vi "TCP Connection Manager (By Reference).vi"(0 "connection manager ref in":T1, 5 "connection in":T3, 7 "index":i32, 9 "method":T5, 11 "error in":errorcluster, 12 "properties in":T2) -> (3 "all properties":T2[](array[typedef]), 4 "connection manager ref out":T1, 6 "connection out":T3, 8 "all connections":T3[](array[typedef]), 10 "number of connections":i32, 14 "properties out":T2, 15 "error out":errorcluster)   [LabVIEW 2015, in "NI STM.lvlib"]
doc: "Copyright 2015, 2016, 2017 National Instruments Corporation\n\nLicensed under the Apache License, Version 2.0 (the \"License\"); you may not use this file except in compliance with the License.\n\n You may obtain a copy of the License at\n\n http://www.apache.org/licenses/LICENSE-2.0\n\nUnless required by applicable law or agreed to in writing, software distributed under the License is distributed on an \"AS IS\" BASIS, WITHOUT WARRANTIES OR CONDITIONS OF ANY KIND, either express or implied.\n\nSee the License for the specific language governing permissions and limitations under the License."
uses:
  <vilib>/NI/STM/NI STM.lvlib
  <vilib>/NI/STM/Connection Manager/TCP/TCP Connection Method.ctl
  <vilib>/NI/STM/TCP/TCP Connection Info.ctl
  <vilib>/NI/STM/SubVIs/MetaDataElement.ctl
  <vilib>/NI/STM/Connection Manager/TCP/TCP Connection Properties.ctl
  <vilib>/NI/STM/Connection Manager/TCP/Advanced/TCP Connection Manager Reference.ctl
  <vilib>/NI/STM/Connection Manager/TCP/Advanced/TCP Connection Manager State Variables.ctl
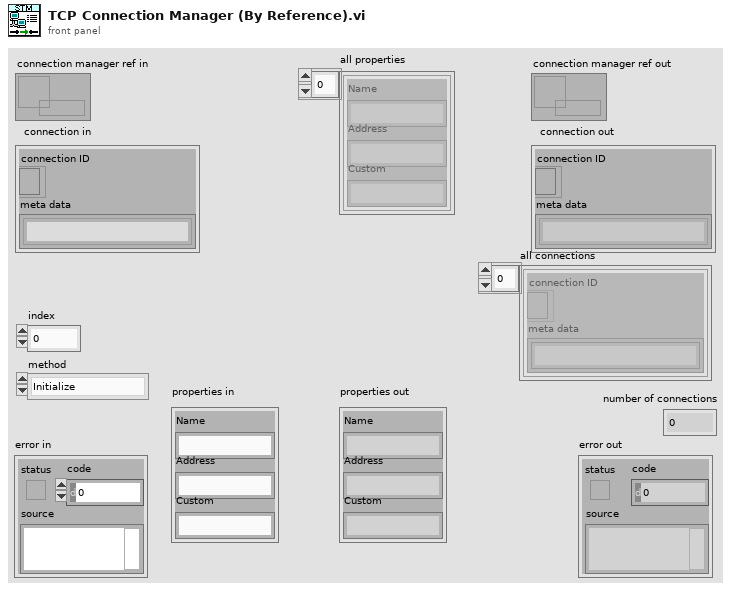
[diagram p1: front panel]
types:
  T1 = typedef "NI STM.lvlib/TCP Connection Manager Reference.ctl" = refnum<data-value>
  T2 = typedef "NI STM.lvlib/TCP Connection Properties.ctl" = cluster{"Name":string, "Address":string, "Custom":string}
  T3 = typedef "NI STM.lvlib/TCP Connection Info.ctl" = cluster{"connection ID":refnum<k5>, "meta data":T4[]}
  T4 = typedef "NI STM.lvlib/MetaDataElement.ctl" = string
  T5 = typedef "NI STM.lvlib/TCP Connection Method.ctl" = enum16{"Initialize", "Add Connection", "Set Properties", "Get Connection(s)", "Remove Connection", "Remove All Connections", "Get Connection Count"}
  T6 = typedef "NI STM.lvlib/TCP Connection Manager State Variables.ctl" = cluster{"Connections":T3[], "Properties":T2[]}
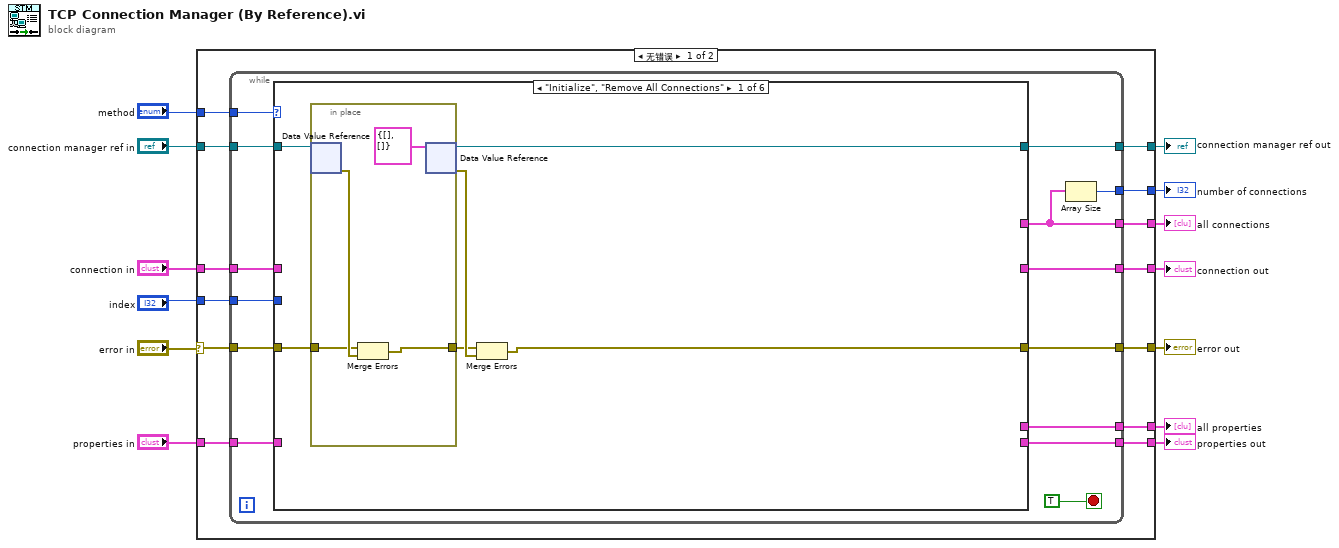
[diagram p0: block diagram]
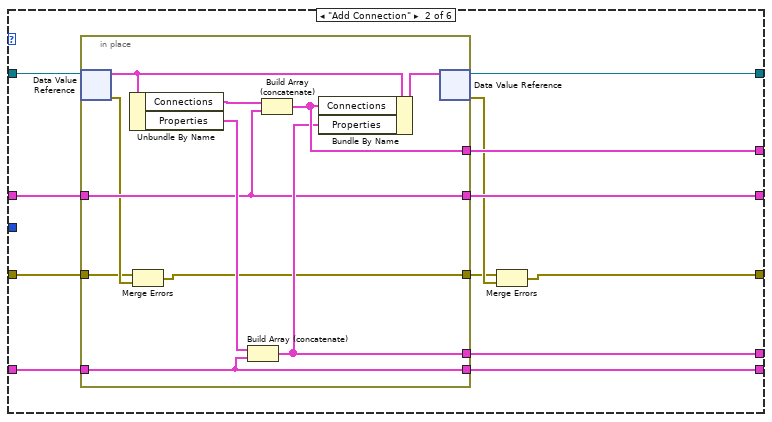
[diagram p2: hidden frame]
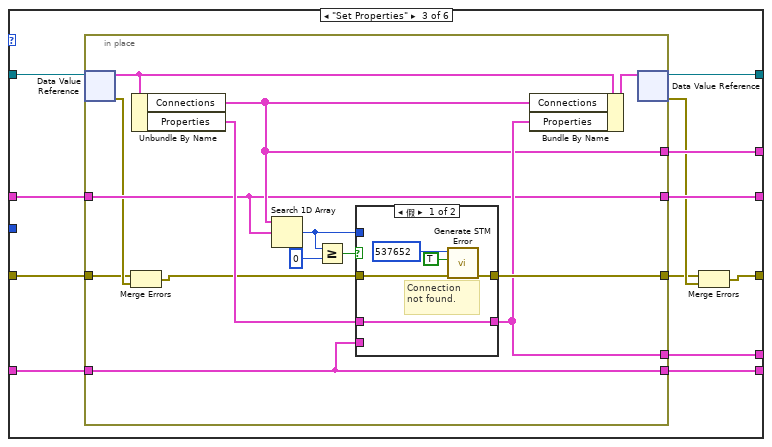
[diagram p3: hidden frame]
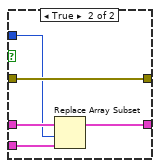
[diagram p4: hidden frame]
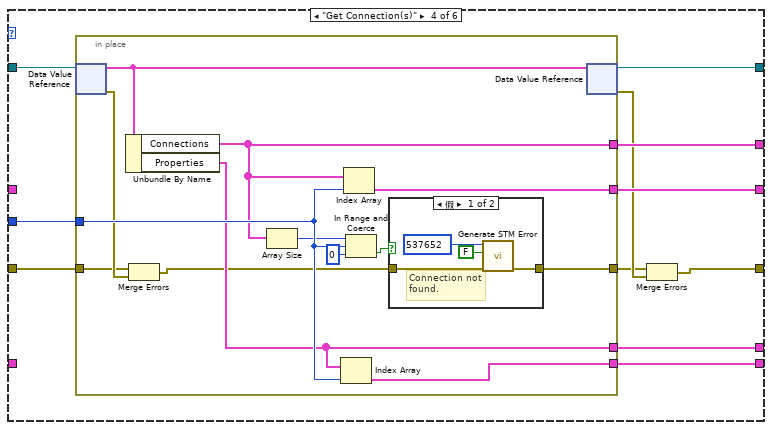
[diagram p5: hidden frame]
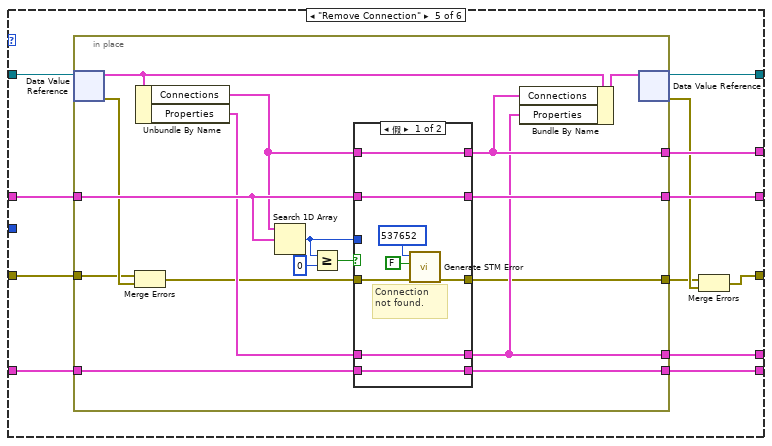
[diagram p7: hidden frame]
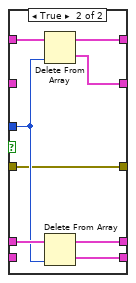
[diagram p8: hidden frame]
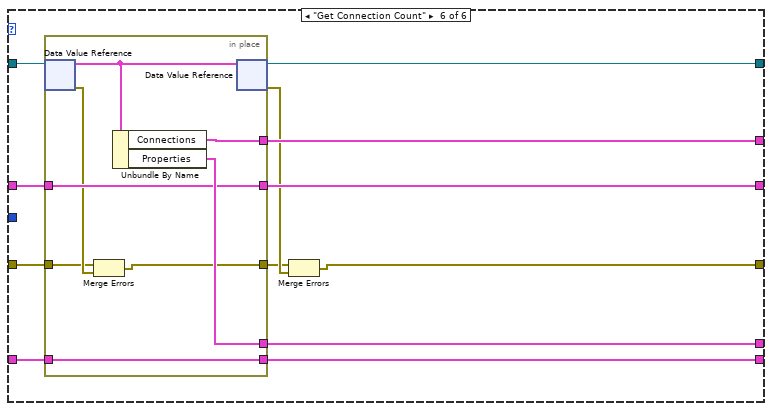
[diagram p9: hidden frame]
diagram:
  n1 = case shown="无错误" "error in" {
    selector: "error in" -> [w26 w206]
    tunnel: [w25 w206] -> w12
    tunnel: "index" -> [w24 _]
    tunnel: "method" -> [w23 _]
    tunnel: "connection in" -> [w22 w205]
    tunnel: [w21 _] -> w8
    tunnel: [w20 _] -> w7
    tunnel: [w19 w205] -> w6
    tunnel: "properties in" -> [w18 _]
    tunnel: [w15 _] -> w4
    tunnel: [w17 _] -> w3
    tunnel: "connection manager ref in" -> [w16 w204]
    tunnel: [w14 w204] -> w1
    frame No Error {
      n2 = while {
        tunnel: w26 -> [w39]
        tunnel: [w38] -> w25
        tunnel: w24 -> [w37]
        tunnel: w23 -> [w36]
        tunnel: w22 -> [w35]
        tunnel: [w34] -> w21
        tunnel: [w33] -> w20
        tunnel: [w32] -> w19
        tunnel: w18 -> [w31]
        tunnel: [w30] -> w17
        tunnel: w16 -> [w29]
        tunnel: [w28] -> w15
        tunnel: [w27] -> w14
        stop <- TRUE stop-if-true
        n3 = case shown="\"Initialize\", \"Remove All Connections\"" w36 {
          tunnel: w35 -> [_ w61 w79 _ w148 w191]
          tunnel: [_ w62 w81 w115 w150 w194] -> w33
          tunnel: [_ w56 w80 w120 w149 w192] -> w32
          tunnel: [w43 w53 w76 w112 w140 w186] -> w38
          tunnel: w39 -> [w45 w57 w85 w117 w143 w188]
          tunnel: w37 -> [_ _ _ w118 _ _]
          tunnel: w31 -> [_ w59 w83 _ w145 w189]
          tunnel: [_ w60 w84 w114 w147 w193] -> w28
          tunnel: [_ w55 w78 w119 w146 w190] -> w30
          tunnel: w29 -> [w46 w58 w82 w116 w144 w195]
          tunnel: [w41 w51 w74 w110 w139 w184] -> w27
          frame "Initialize", "Remove All Connections" {
            n4 = in-place {
              in-place-border: [w47] -> w42
              in-place-border: w45 -> [w48]
              n5 = in-place-dvr #1(w46) -> (w49:errorcluster)  [unwired: 1 out]
              n6 = Merge Errors(w48, w49) -> (w47:errorcluster)
              n7 = in-place-dvr #1(T6 {"Connections"=[], "Properties"=[]}) -> (w41:T1, w44:errorcluster)
            }
            n8 = Merge Errors(w42, w44) -> (w43:errorcluster)
          }
          frame "Add Connection" {
            n9 = in-place {
              in-place-border: [w69] -> w62
              in-place-border: w61 -> [w67]
              in-place-border: [w68] -> w60
              in-place-border: w59 -> [w66]
              in-place-border: [w63] -> w52
              in-place-border: w57 -> [w64]
              in-place-border: [w67] -> w56
              in-place-border: [w66] -> w55
              n10 = in-place-dvr #2(w58) -> (w72:T6, w65:errorcluster)
              n11 = Unbundle By Name(w72) -> ("Connections"=w73:T3[], "Properties"=w71:T2[])
              n12 = Merge Errors(w64, w65) -> (w63:errorcluster)
              n13 = Build Array (concatenate)(w71, w66) -> (w68:T2[])
              n14 = Build Array (concatenate)(w73, w67) -> (w69:T3[])
              n15 = Bundle By Name(cluster=w72, "Connections"=w69, "Properties"=w68) -> (w70:T6)
              n16 = in-place-dvr #2(w70) -> (w51:T1, w54:errorcluster)
            }
            n17 = Merge Errors(w52, w54) -> (w53:errorcluster)
          }
          frame "Set Properties" {
            n18 = in-place {
              in-place-border: w85 -> [w87]
              in-place-border: [w97] -> w75
              in-place-border: [w93] -> w84
              in-place-border: w83 -> [w90]
              in-place-border: [w91] -> w81
              in-place-border: [w89] -> w80
              in-place-border: w79 -> [w89]
              in-place-border: [w90] -> w78
              n19 = in-place-dvr #3(w82) -> (w94:T6, w88:errorcluster)
              n20 = Merge Errors(w87, w88) -> (w86:errorcluster)
              n21 = Unbundle By Name(w94) -> ("Connections"=w91:T3[], "Properties"=w95:T2[])
              n22 = Search 1D Array(1D array=w91, element=w89) -> (index of element=w96:i32)  [unwired: 1 out]
              n23 = Greater Or Equal?(x=w96, y=0) -> (x >= y?=w98:bool)
              n24 = case shown="假" w98 {
                tunnel: w86 -> [w101 w109]
                tunnel: [w100 w109] -> w97
                tunnel: w95 -> [w104 w108]
                tunnel: w96 -> [_ w107]
                tunnel: w90 -> [_ w106]
                tunnel: [w104 w105] -> w93
                frame False {
                  # "Connection not found."
                  n25 = call <vilib>:"Generate STM Error.vi"("error in"=w101, "status (T)"=TRUE, "code"=537652) -> ("error out"=w100:errorcluster)  [unwired: 8 in]
                }
                frame True {
                  n26 = Replace Array Subset(array=w108, new element=w106, index=w107) -> (w105:T2[])
                }
              }
              n27 = Bundle By Name(cluster=w94, "Connections"=w91, "Properties"=w93) -> (w92:T6)
              n28 = in-place-dvr #3(w92) -> (w74:T1, w77:errorcluster)
            }
            n29 = Merge Errors(w75, w77) -> (w76:errorcluster)
          }
          frame "Get Connection(s)" {
            n30 = in-place {
              in-place-border: [w133] -> w120
              in-place-border: [w132] -> w119
              in-place-border: w118 -> [w131]
              in-place-border: w117 -> [w122]
              in-place-border: [w127] -> w111
              in-place-border: [w125] -> w115
              in-place-border: [w124] -> w114
              n31 = in-place-dvr #4(w116) -> (w126:T6, w123:errorcluster)
              n32 = Unbundle By Name(w126) -> ("Connections"=w125:T3[], "Properties"=w124:T2[])
              n33 = Merge Errors(w122, w123) -> (w121:errorcluster)
              n34 = Array Size(array=w125) -> (size(s)=w130:i32)
              n35 = Index Array(array=w124, index=w131) -> (element=w132:T2)
              n36 = Index Array(array=w125, index=w131) -> (element=w133:T3)
              n37 = In Range and Coerce(upper limit=w130, x=w131, lower limit=0) -> (In Range?=w129:bool)  [unwired: 1 out]
              n38 = case shown="假" w129 {
                tunnel: w121 -> [w135 w138]
                tunnel: [w134 w138] -> w127
                frame False {
                  # "Connection not found."
                  n39 = call <vilib>:"Generate STM Error.vi"("error in"=w135, "status (T)"=FALSE, "code"=537652) -> ("error out"=w134:errorcluster)  [unwired: 8 in]
                }
                frame True {
                }
              }
              n40 = in-place-dvr #4(w126) -> (w110:T1, w113:errorcluster)
            }
            n41 = Merge Errors(w111, w113) -> (w112:errorcluster)
          }
          frame "Remove Connection" {
            n42 = in-place {
              in-place-border: [w157] -> w150
              in-place-border: [w164] -> w149
              in-place-border: w148 -> [w163]
              in-place-border: [w156] -> w147
              in-place-border: [w162] -> w146
              in-place-border: w145 -> [w161]
              in-place-border: w143 -> [w153]
              in-place-border: [w151] -> w141
              n43 = in-place-dvr #5(w144) -> (w158:T6, w154:errorcluster)
              n44 = Merge Errors(w153, w154) -> (w152:errorcluster)
              n45 = Unbundle By Name(w158) -> ("Connections"=w160:T3[], "Properties"=w159:T2[])
              n46 = Search 1D Array(1D array=w160, element=w163) -> (index of element=w167:i32)  [unwired: 1 out]
              n47 = Greater Or Equal?(x=w167, y=0) -> (x >= y?=w165:bool)
              n48 = case shown="假" w165 {
                tunnel: w160 -> [w175 w182]
                tunnel: w167 -> [_ w179]
                tunnel: [w175 w183] -> w157
                tunnel: [w174 w177] -> w164
                tunnel: [w168 w176] -> w151
                tunnel: w152 -> [w169 w176]
                tunnel: w163 -> [w174 _]
                tunnel: w159 -> [w173 w181]
                tunnel: [w173 w180] -> w156
                tunnel: [w172 w178] -> w162
                tunnel: w161 -> [w172 _]
                frame False {
                  # "Connection not found."
                  n49 = call <vilib>:"Generate STM Error.vi"("error in"=w169, "status (T)"=FALSE, "code"=537652) -> ("error out"=w168:errorcluster)  [unwired: 8 in]
                }
                frame True {
                  n50 = Delete From Array(array=w182, index=w179) -> (deleted portion=w177:T3, array with subset deleted=w183:T3[])  [unwired: 1 in]
                  n51 = Delete From Array(array=w181, index=w179) -> (deleted portion=w178:T2, array with subset deleted=w180:T2[])  [unwired: 1 in]
                }
              }
              n52 = Bundle By Name(cluster=w158, "Connections"=w157, "Properties"=w156) -> (w155:T6)
              n53 = in-place-dvr #5(w155) -> (w139:T1, w142:errorcluster)
            }
            n54 = Merge Errors(w141, w142) -> (w140:errorcluster)
          }
          frame "Get Connection Count" {
            n55 = in-place {
              in-place-border: [w202] -> w194
              in-place-border: [w201] -> w193
              in-place-border: [w200] -> w192
              in-place-border: w191 -> [w200]
              in-place-border: [w199] -> w190
              in-place-border: w189 -> [w199]
              in-place-border: [w196] -> w185
              in-place-border: w188 -> [w197]
              n56 = in-place-dvr #6(w195) -> (w203:T6, w198:errorcluster)
              n57 = Merge Errors(w197, w198) -> (w196:errorcluster)
              n58 = Unbundle By Name(w203) -> ("Connections"=w202:T3[], "Properties"=w201:T2[])
              n59 = in-place-dvr #6(w203) -> (w184:T1, w187:errorcluster)
            }
            n60 = Merge Errors(w185, w187) -> (w186:errorcluster)
          }
        }
        n61 = Array Size(array=w33) -> (size(s)=w34:i32)
      }
    }
    frame Error {
    }
  }
  "error out" <- w12
  "number of connections" <- w8
  "all connections" <- w7
  "connection out" <- w6
  "all properties" <- w4
  "properties out" <- w3
  "connection manager ref out" <- w1
